vi "Get Attr Dict.vi"(7 "Tree ID":string, 8 "Error In":errorcluster, 11 "Tree Manager":T1) -> (0 "Error Out":errorcluster, 1 "Attributes Dictionary":variant, 3 "Tree Manager":T1)   [LabVIEW 2016, in "Tree Manager.lvclass"]
doc: "Get variant attribute dictionary of the Tree. \n\n<b>WARNING</b> Any modifications of this dictionary are not reflected in the Tree until it is set back."
uses:
  Tree Manager.lvclass
  Typedefs/Session Handle.ctl
  Tree Manager.lvclass/Tree Manager.ctl
  Typedefs/Tree.ctl
  <vilib>/Utility/error.llb/Error Cluster From Error Code.vi
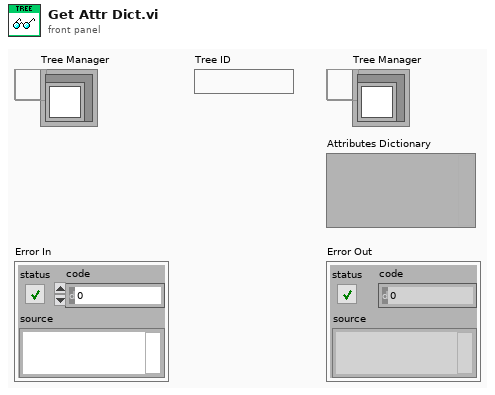
[diagram p1: front panel]
types:
  T1 = typedef "Tree Manager.lvclass/Session Handle.ctl" = refnum<data-value>
  T2 = typedef "Tree Manager.lvclass/Tree.ctl" = cluster{"Unique ID":string, "Parent ID":string, "Child IDs":string[], "Data":variant, "Name":string}
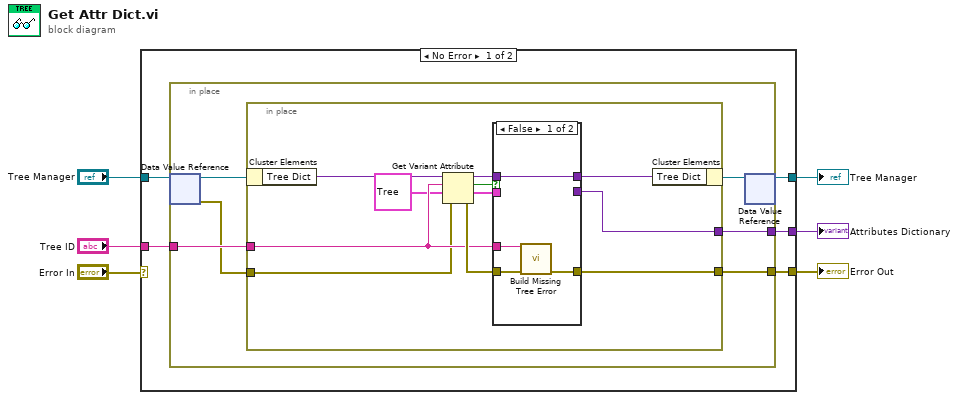
[diagram p0: block diagram]
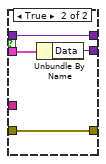
[diagram p2: hidden frame]
diagram:
  n1 = case shown="No Error" "Error In" {
    selector: "Error In" -> [_ w37]
    tunnel: "Tree Manager" -> [w11 w38]
    tunnel: [w10 w38] -> w5
    tunnel: [w9 w37] -> w3
    tunnel: "Tree ID" -> [w8 _]
    tunnel: [w7 _] -> w1
    frame No Error {
      n2 = in-place {
        in-place-border: [w16] -> w9
        in-place-border: w8 -> [w14]
        in-place-border: [w13] -> w7
        n3 = in-place-dvr #1(w11) -> (w17:refnum<class "Tree Manager.lvclass">, w12:errorcluster)
        n4 = in-place {
          in-place-border: [w20] -> w16
          in-place-border: w12 -> [w21]
          in-place-border: w14 -> [w22]
          in-place-border: [w19] -> w13
          n5 = in-place-cluster #2(w17) -> ("Tree Dict"=w24:variant)
          n6 = Get Variant Attribute(Variant=w24, name=w22, default value (empty Variant)=T2 {"Unique ID"="", "Parent ID"="", "Child IDs"=[], "Data"=variant, "Name"=""} ("Cluster of class private data"), error in=w21) -> (duplicate Variant=w27:variant, found=w25:bool, value=w26:T2, error out=w28:errorcluster)
          n7 = case shown="False" w25 {
            tunnel: w26 -> [_ w34]
            tunnel: w27 -> [w32 w36]
            tunnel: w28 -> [w31 w35]
            tunnel: [w30 w35] -> w20
            tunnel: [w32 w36] -> w23
            tunnel: w22 -> [w29 _]
            tunnel: [_ w33] -> w19
            frame False {
              n8 = call "Build Missing Tree Error.vi"("Unique ID"=w29, "Error In"=w31) -> ("Error Out"=w30:errorcluster)  [unwired: 13 in]
            }
            frame True {
              n9 = Unbundle By Name(w34) -> ("Data"=w33:variant)
            }
          }
          n10 = in-place-cluster #2("Tree Dict"=w23) -> (w15:refnum<class "Tree Manager.lvclass">)
        }
        n11 = in-place-dvr #1(w15) -> (w10:T1)  [unwired: 1 out]
      }
    }
    frame Error {
    }
  }
  "Tree Manager" <- w5
  "Error Out" <- w3
  "Attributes Dictionary" <- w1
